vi "Find DAQ Devices.vi"(8 "Error In":errorcluster, 9 "Search Term":string, 10 "Return":enum16{"Device ID", "Product", "Serial Number"}(ring), 11 "Search By":enum16{"Device ID", "Product", "Serial Number"}(ring)) -> (0 "Error Out":errorcluster, 1 "All Connected Devices":string[][](table), 2 "Returned Element":string, 4 "All Device IDs":tag[](array[tag]), 6 "All Serial Numbers":u32[](array[numeric]))   [LabVIEW 2013]
doc: "This VI returns information on all DAQ devices connected to the development computer. \n\nIf you do not wire any of the search inputs it will not return an element. It will, however, return the list of connected devices and serial numbers and a table of all the devices connected."
uses:
  <resource>/objmgr/daqmx.rc
panel:
  # "Input"
  # "Output"
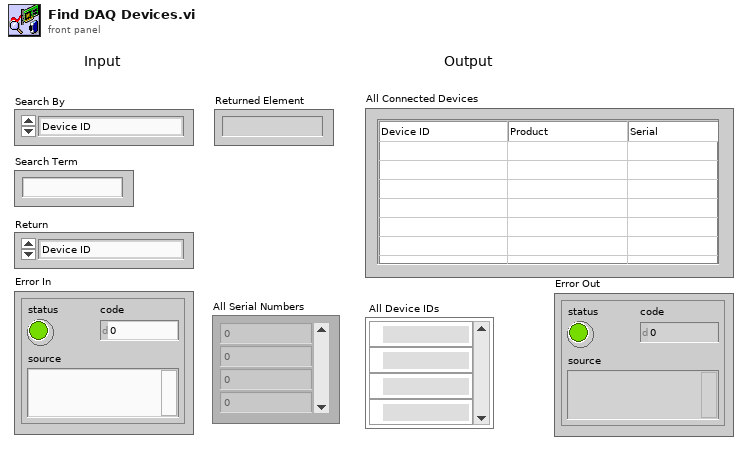
[diagram p1: front panel]
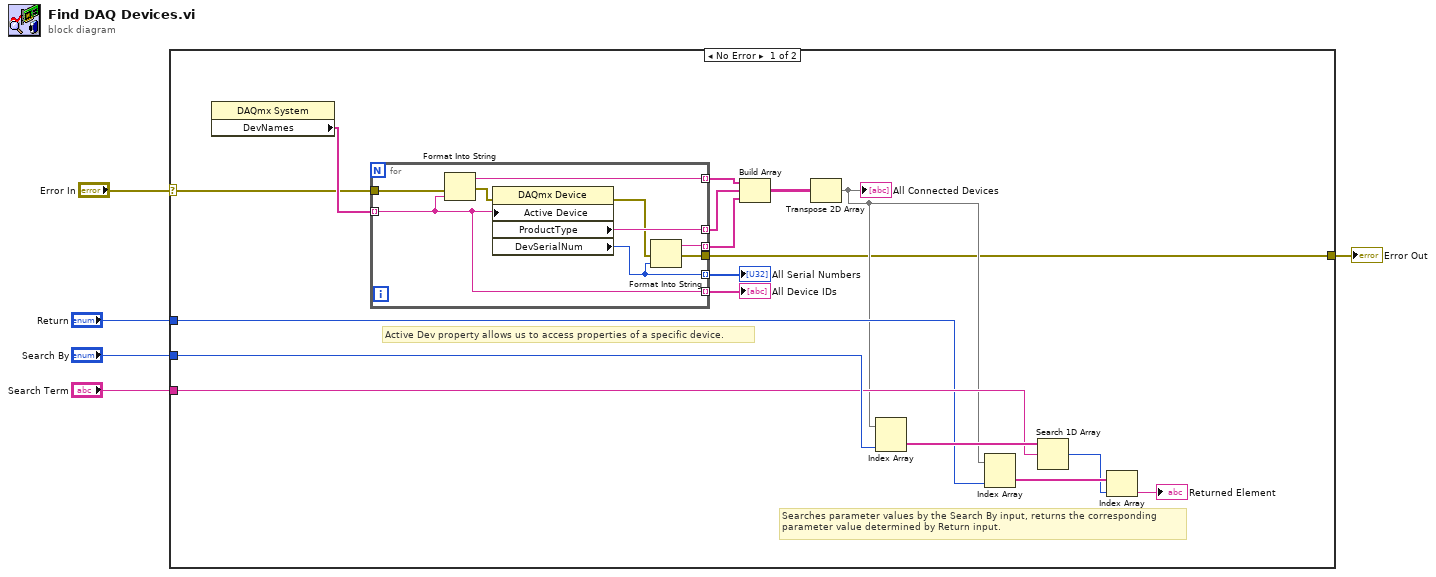
[diagram p0: block diagram]
diagram:
  n1 = case shown="No Error" "Error In" {
    selector: "Error In" -> [w7 w32]
    tunnel: "Search By" -> [w22 _]
    tunnel: "Search Term" -> [w20 _]
    tunnel: "Return" -> [w19 _]
    tunnel: [w6 w32] -> w1
    frame No Error {
      # "Active Dev property allows us to access properties of a specific device."
      # "Searches parameter values by the Search By input, returns the corresponding\nparameter value determined by Return input."
      n2 = property class="DAQmx System"() -> ("DevNames"=w9:tag[])  [unwired: 2 in, 2 out]
      n3 = for {
        tunnel: w9 -> [w28] mode=indexing
        tunnel: [w31] -> w11 mode=indexing
        tunnel: [w27] -> w10 mode=indexing
        tunnel: [w30] -> w12 mode=indexing
        tunnel: [w29] -> w13 mode=indexing
        tunnel: [w28] -> w15 mode=indexing
        tunnel: [w24] -> w6
        tunnel: w7 -> [w23]
        n4 = Format Into String(error in=w23, w28) -> (resulting string=w30:string, error out=w26:errorcluster)  [unwired: 2 in]
        n5 = property class="DAQmx Device"(error in=w26, "Active Device"=w28) -> (error out=w25:errorcluster, "ProductType"=w31:string, "DevSerialNum"=w27:u32)  [unwired: 1 in, 1 out]
        n6 = Format Into String(error in=w25, w27) -> (resulting string=w29:string, error out=w24:errorcluster)  [unwired: 2 in]
      }
      "All Serial Numbers" <- w10
      "All Device IDs" <- w15
      n7 = Build Array(w12, w11, w13) -> (w14:string[][])
      n8 = Transpose 2D Array(2D array=w14) -> (transposed array=w8:string[][])
      "All Connected Devices" <- w8
      n9 = Index Array(array=w8, index (col)=w22) -> (element=w21:string[])  [unwired: 1 in]
      n10 = Index Array(array=w8, index (col)=w19) -> (element=w18:string[])  [unwired: 1 in]
      n11 = Search 1D Array(1D array=w21, element=w20) -> (index of element=w17:i32)  [unwired: 1 in]
      n12 = Index Array(array=w18, index=w17) -> (element=→"Returned Element":string)
    }
    frame Error {
    }
  }
  "Error Out" <- w1
